vi "Create Plugin Timing Group.vi"(5 "Plugin ID":i32, 7 "Plugin Timing":refnum<class "Timing.lvclass">, 8 "Async Tx":refnum<class "Transfer Group Timing.lvclass">[](array[class]), 9 "Async Rx":refnum<class "Transfer Group Timing.lvclass">[](array[class]), 10 "Inline Tx":refnum<class "Transfer Group Timing.lvclass">[](array[class]), 11 "Inline Rx":refnum<class "Transfer Group Timing.lvclass">[](array[class])) -> (3 "Plugin Timing Group":refnum<class "Plugin Timing Group.lvclass">)   [LabVIEW 2017, in "DSF Core.lvlib" / "Plugin Timing Group.lvclass"]
uses:
  Plugin Timing Group.lvclass
  Transfer Group Timing.lvclass
  Timing.lvclass
  Plugin Timing Group.lvclass/Plugin Timing Group.ctl
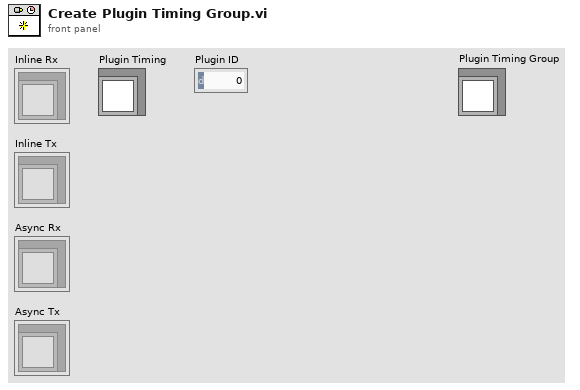
[diagram p1: front panel]
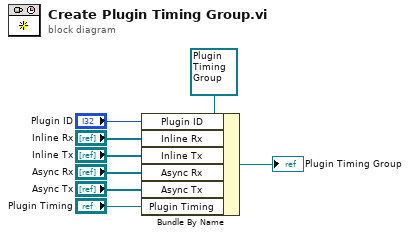
[diagram p0: block diagram]
diagram:
  n1 = Bundle By Name(cluster=refnum<class "Plugin Timing Group.lvclass"> refnum ("Plugin Timing in"), "Plugin ID"="Plugin ID", "Inline Rx"="Inline Rx", "Inline Tx"="Inline Tx", "Async Rx"="Async Rx", "Async Tx"="Async Tx", "Plugin Timing"="Plugin Timing") -> (→"Plugin Timing Group":refnum<class "Plugin Timing Group.lvclass">)
